vi "Error Channels Write Array.vi"(8 "error in":errorcluster, 10 "Error Channels STS":i32[](array[numeric]), 11 "Chiller in":refnum<class "Chiller.lvclass">) -> (0 "error out":errorcluster, 3 "Chiller out":refnum<class "Chiller.lvclass">)   [LabVIEW 2023, in "Chiller.lvclass"]
uses:
  Chiller.lvclass
  Low Level Capabilities/Error Channels/Error Channels.lvclass
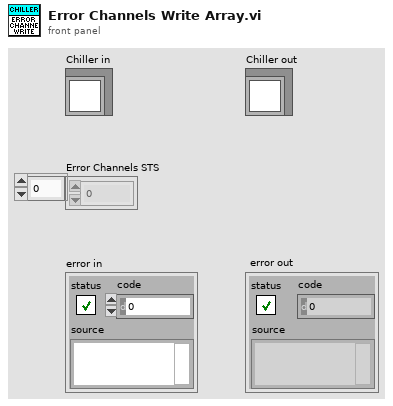
[diagram p1: front panel]
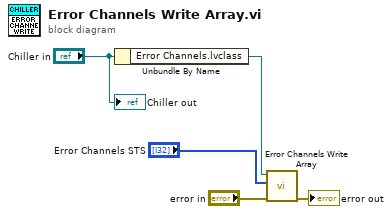
[diagram p0: block diagram]
diagram:
  n1 = Unbundle By Name("Chiller in") -> ("Error Channels.lvclass"=w5:refnum<class "Error Channels.lvclass">)
  n2 = call-dynamic "Error Channels Write Array.vi"("error in (no error)"="error in", "Error Channels STS"="Error Channels STS", "Error Channels in"=w5) -> ("error out"=→"error out":errorcluster)  [unwired: 7 in, 1 out]
  "Chiller out" <- "Chiller in"
